vi "conversational read signals.vi"(0 "Serial Port":refnum<visa-resource-name>, 5 "Max time (ms)":u32=2000, 7 "signals":enum16{"signal 1", "signals 1 and 2"}(ring)=enum."signals 1 and 2", 9 "data points":u8=5, 11 "i":i32) -> (3 "Serial Port":refnum<visa-resource-name>, 4 "Time out":bool, 6 "correct command":bool, 8 "run done":bool, 10 "signal 1":dbl[](array[numeric]) format="%.2f", 14 "emptied buffer":bool, 15 "signal 2":dbl[](array[numeric]) format="%.2f")   [LabVIEW 2012]
panel:
  out "channel":u8=2
  out "return string":string
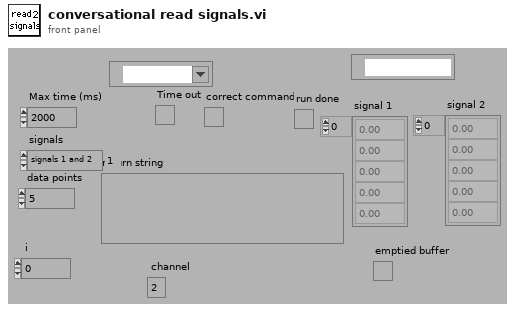
[diagram p1: front panel]
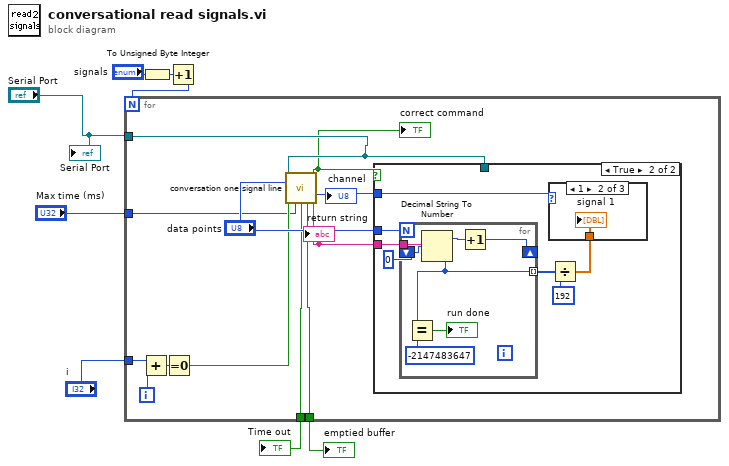
[diagram p0: block diagram]
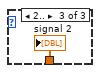
[diagram p4: hidden frame]
diagram:
  n1 = To Unsigned Byte Integer(number="signals") -> (unsigned 8bit integer=w7:u8)
  n2 = Increment(x=w7) -> (x+1=w6:u8)
  n3 = for {
    N: w6 -> [_]
    tunnel: "Serial Port" -> [w15]
    tunnel: "i" -> [w18]
    tunnel: "Max time (ms)" -> [w12]
    tunnel: [w11] -> w3
    tunnel: [w10] -> w2
    i -> [w17]
    n4 = Add(x=w18, y=w17) -> (x+y=w16:i32)
    n5 = Equal To 0?(x=w16) -> (x = 0?=w13:bool)
    n6 = call "conversation one signal line.vi"("Serial Port"=w15, "data points"="data points", "first"=w13, "Max time (ms)"=w12) -> ("correct command"=w9:bool, "channel"=w20:u8, "Time out"=w10:bool, "emptied buffer"=w11:bool, "return string"=w19:string)  [unwired: 4 in, 3 out]
    "channel" <- w20
    "return string" <- w19
    "correct command" <- w9
    n7 = case shown="True" w9 {
      tunnel: w15 -> [_ _]
      tunnel: w20 -> [_ w25]
      tunnel: w19 -> [_ w26]
      tunnel: "data points" -> [_ w24]
      frame False {
      }
      frame True {
        n8 = for {
          N: w24 -> [_]
          tunnel: w26 -> [w36]
          shift-right: [w33] -> _
          shift-left: 0 -> [w35]
          tunnel: [w30] -> w22 mode=indexing
          n9 = Decimal String To Number(string=w36, offset=w35) -> (offset past number=w34:i32, number=w30:i32)  [unwired: 1 in]
          n10 = Equal?(x=w30, y=-2147483647) -> (x = y?=→"run done":bool)
          n11 = Increment(x=w34) -> (x+1=w33:i32)
        }
        n12 = Divide(x=w22, y=192) -> (x/y=w23:dbl[])
        n13 = case shown="1" w25 {
          tunnel: w23 -> [_ w28 w29]
          frame ..0 {
          }
          frame 1 {
            "signal 1" <- w28
          }
          frame 2.. {
            "signal 2" <- w29
          }
        }
      }
    }
  }
  "emptied buffer" <- w3
  "Time out" <- w2
  "Serial Port" <- "Serial Port"
